vi "Login.vi"() -> (3 "Login Password 2":string, 4 "Cancle":bool, 5 "Enter":bool)   [LabVIEW 2014, in "Master.lvclass"]
uses:
  Master.lvclass
panel:
  in  "Cancel":bool caption="Cancle"
  in  "Enter":bool
  in  "Enter Admin Password":string
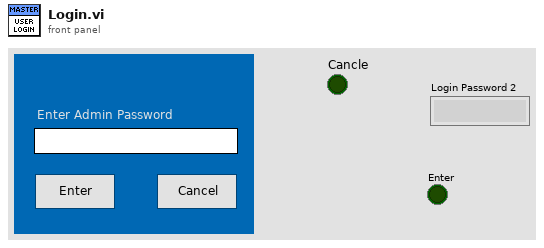
[diagram p1: front panel]
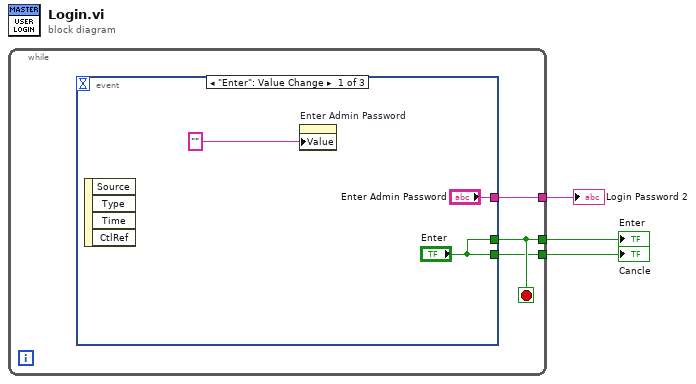
[diagram p0: block diagram]
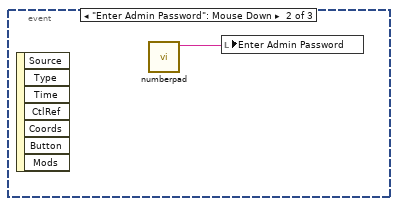
[diagram p2: hidden frame]
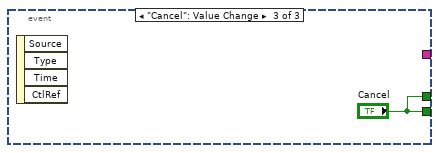
[diagram p3: hidden frame]
diagram:
  n1 = while {
    tunnel: [w6] -> w3
    tunnel: [w5] -> w2
    tunnel: [w4] -> w1
    stop <- w5 stop-if-true
    n2 = event shown="[0] \"Enter\": Value Change" {
      selector: _ -> [_ _ _]
      dyn-events: _ -> [_ _ _]
      timeout: _ -> [_ _ _]
      tunnel: ["Enter" _ "Cancel"] -> w4
      tunnel: ["Enter Admin Password" _ _] -> w6
      tunnel: ["Enter" _ "Cancel"] -> w5
      event "Enter": Value Change {
        n3 = event-data() -> ()  [unwired: 1 in, 4 out]
        n4 = property on="Enter Admin Password" class="Str"("Value"="" ("Login Password")) -> ()  [unwired: 2 in, 2 out]
      }
      event "Enter Admin Password": Mouse Down {
        n5 = event-data() -> ()  [unwired: 1 in, 7 out]
        n6 = call "numberpad.vi"() -> ("String"=w10:string)  [unwired: 11 in]
        n7 = local write "Enter Admin Password"(w10) -> ()
      }
      event "Cancel": Value Change {
        n8 = event-data() -> ()  [unwired: 1 in, 4 out]
      }
    }
  }
  "Login Password 2" <- w3
  "Enter" <- w2
  "Cancle" <- w1
